vi "Pfeiffer Vacuum Turbo Run up time.vi"(7 "Adress of unit":u16=1 min=1 max=999 step=1, 8 "error in (no error)":errorcluster, 11 "COM Port Name in":refnum<visa-resource-name>="COM1") -> (0 "error out":errorcluster {"code" format="%.0x"}, 3 "response (data)":string)   [LabVIEW 2021]
doc: "This VI is an example of how to use the Pfeiffer Vacuum subVIs programmatically. This VI first initializes the instrument, takes measurements, then closes the instrument."
uses:
  <instrlib>/Pfeiffer Vacuum/Public/Turbopumps/PV Run-up time - Cluster.ctl
  <instrlib>/Pfeiffer Vacuum/Pfeiffer Vacuum.lvlib
panel:
  in  "PV Run-up time - Cluster":T1={"Parameter"=0, "Parameter\nread only<->describe"=FALSE, "Run-up time monitoring\noff     <----->     on"=TRUE, "maximum run-up\ntime [min]"=15, "speed switchpoint\n1 + 2  [%]"=80, "configuration rotation\nspeed switchpoint"=0} {"configuration rotation\nspeed switchpoint" items=["rotation speed switchpoint 1 ", "rotation speed switchpoint 1 & 2"]; "Parameter" items=["Run-up time monitoring [off/on] (004)", "run-up time [min] (700)", "speed switchpoint 1 [%] (701)", "speed switchpoint 2 [%] (719)", "configuration rotation speed switchpoint (017)"]; "speed switchpoint\n1 + 2  [%]" min=40 max=98 step=1; "maximum run-up\ntime [min]" min=1 max=120 step=1}
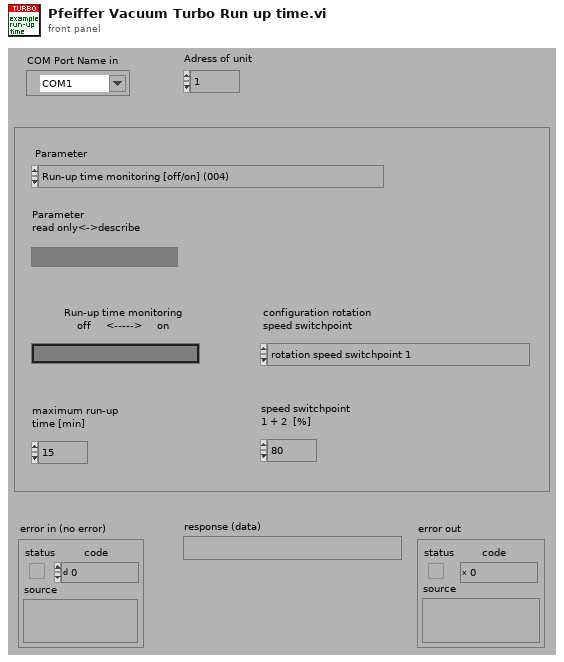
[diagram p1: front panel]
types:
  T1 = typedef "Pfeiffer Vacuum.lvlib/PV Run-up time - Cluster.ctl" = cluster{"Parameter":u16, "Parameter\nread only<->describe":bool, "Run-up time monitoring\noff     <----->     on":bool, "maximum run-up\ntime [min]":u16, "speed switchpoint\n1 + 2  [%]":u16, "configuration rotation\nspeed switchpoint":u16}
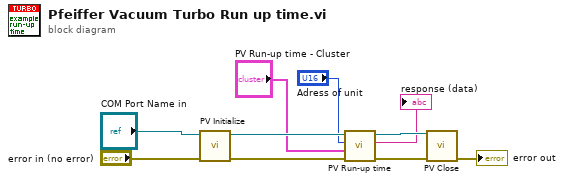
[diagram p0: block diagram]
diagram:
  n1 = call <instrlib>:"PV Initialize.vi"("error in (no error)"="error in (no error)", "VISA session in"="COM Port Name in") -> ("error out"=w8:errorcluster, "VISA session out"=w9:refnum<visa-resource-name>)  [unwired: 8 in]
  n2 = call <instrlib>:"PV Run-up time.vi"("error in (no error)"=w8, "PV Run-up time - Cluster"="PV Run-up time - Cluster", "Adress of unit"="Adress of unit", "VISA session"=w9) -> ("error out"=w5:errorcluster, "response (data)"=→"response (data)":string, "dup VISA session"=w6:refnum<visa-resource-name>)  [unwired: 5 in]
  n3 = call <instrlib>:"PV Close.vi"("VISA session"=w6, "error in (no error)"=w5) -> ("error out"=→"error out":errorcluster)  [unwired: 13 in]
